vi "Editor UI.vi"(8 "error in (no error)":errorcluster, 11 "Entity Editor in":refnum<class "Entity Editor.lvclass">) -> (0 "error out":errorcluster, 3 "Entity Editor out":refnum<class "Entity Editor.lvclass">)   [LabVIEW 2020, in "Conditum-Tools.lvlib" / "Entity Editor.lvclass"]
uses:
  Entity Editor.lvclass
  Conditum/Columns/Type/Type.lvclass
  Conditum/Entity/Entity.lvclass
  ColumnPanel/ColumnPanel.lvclass
  C:/Program Files (x86)/National Instruments/LabVIEW 2020/vi.lib/IlluminatedG/IG OOPanel/OOPanel/ArrayPanel/ArrayPanel.lvclass
  Conditum/Columns/Type/Type.lvclass/Type.ctl
  <vilib>/IlluminatedG/IG OOPanel/OOPanel/ArrayManager/ArrayManager.lvclass
  2443108f-0f49-4029-b3c0-d61e9c764f54.vi
  1c4234d0-757c-494a-9175-61bb4fd4687c.vi
  <vilib>/Utility/LVClass/Get LV Class Name.vi
  <vilib>/Comparison/Equal/Equal Functor/Equal Functor.lvclass
panel:
  in  "Reset Entity":bool
  in  "Save Entity":bool
  in  "Fields":i32(listbox)
  out "Definition":refnum<class "Type.lvclass">[](array[class])
  out "Target Entity Paths":path[](array[path])
  in  "Refresh Targets":bool
  in  "Target":string(combo)
  in  "Refresh Projects":bool
  in  "New Entity":bool
  in  "Remove Field":bool
  in  "Add Field":bool
  in  "Entities":i32(listbox)
  in  "Project":string(combo)
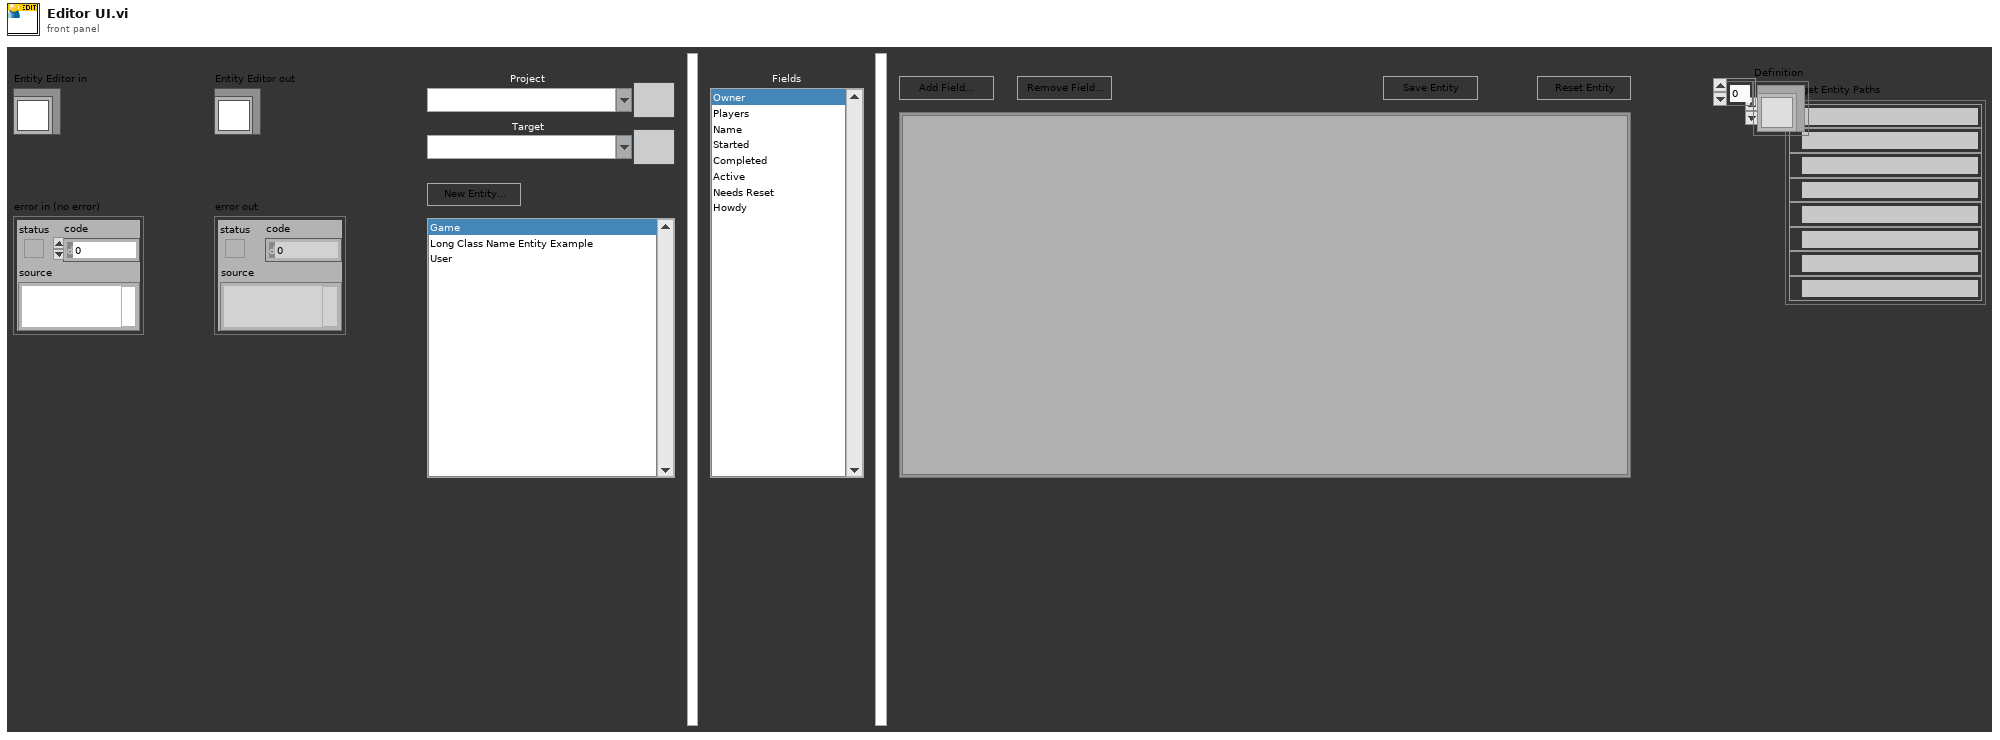
[diagram p1: front panel]
types:
  T1 = typedef "Conditum.lvlib/Field Type.ctl" = enum16{"None", "ID", "Boolean", "Integer", "Double", "Timestamp", "String", "Text", "Entity"}
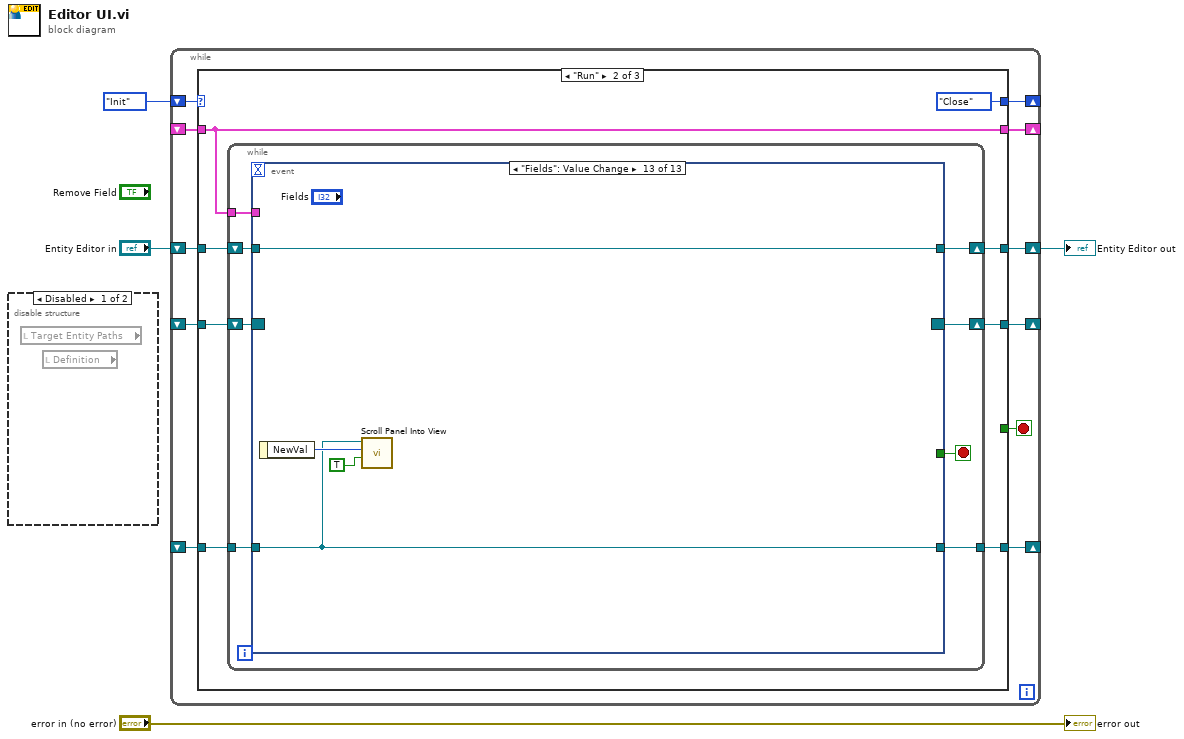
[diagram p0: block diagram]
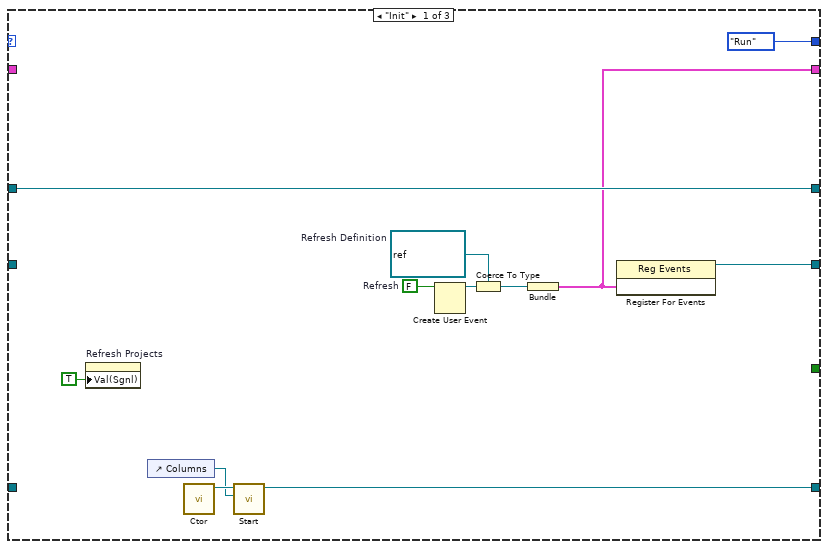
[diagram p3: hidden frame]
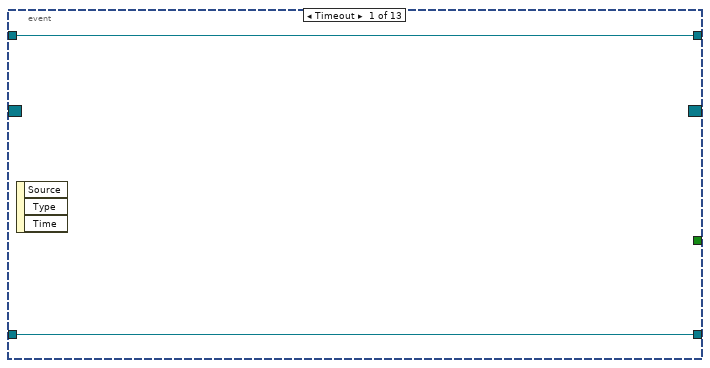
[diagram p4: hidden frame]
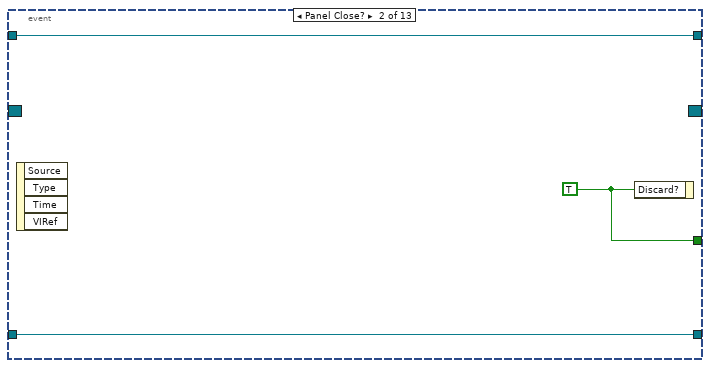
[diagram p5: hidden frame]
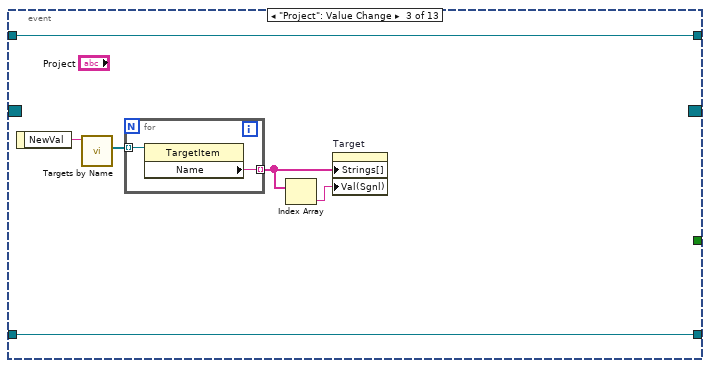
[diagram p6: hidden frame]
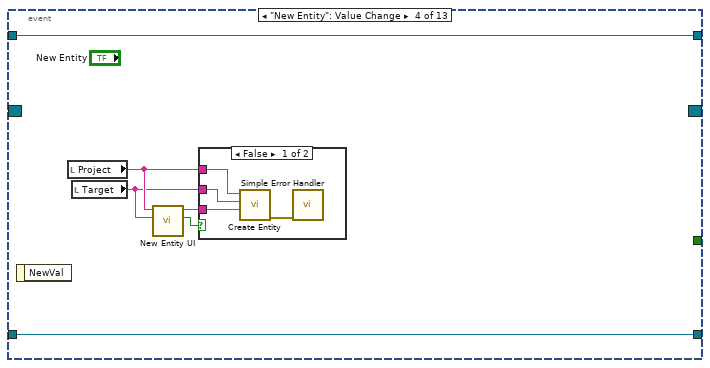
[diagram p7: hidden frame]
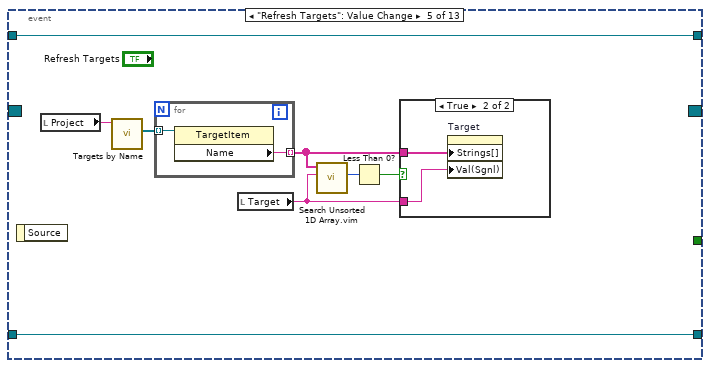
[diagram p9: hidden frame]
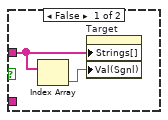
[diagram p10: hidden frame]
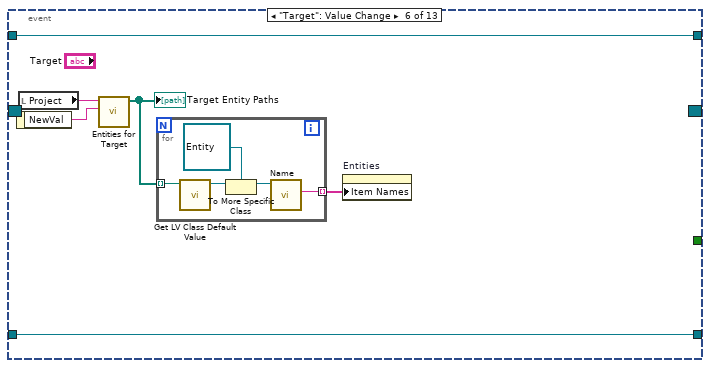
[diagram p11: hidden frame]
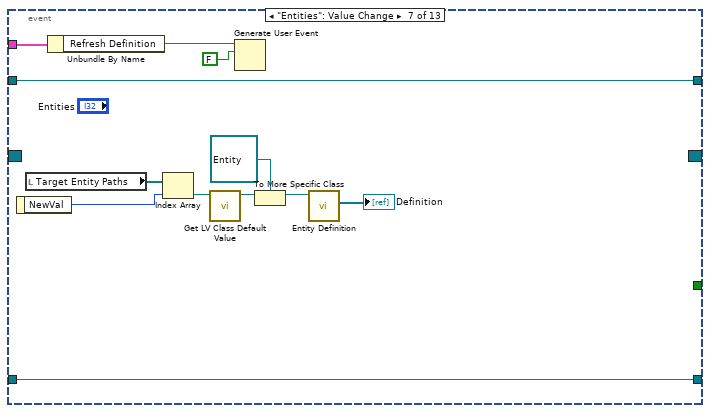
[diagram p12: hidden frame]
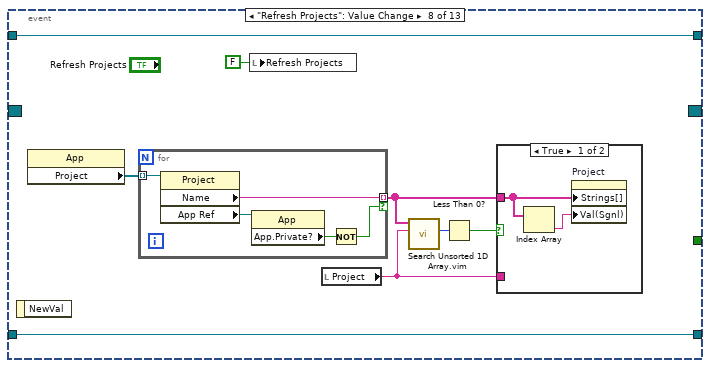
[diagram p13: hidden frame]
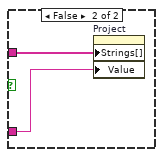
[diagram p14: hidden frame]
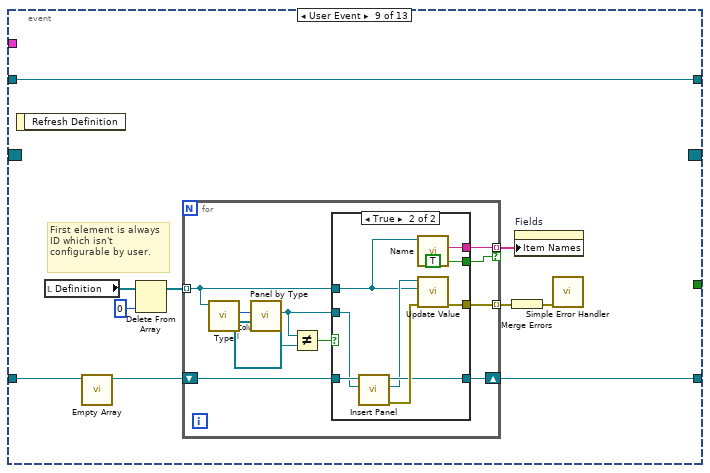
[diagram p15: hidden frame]
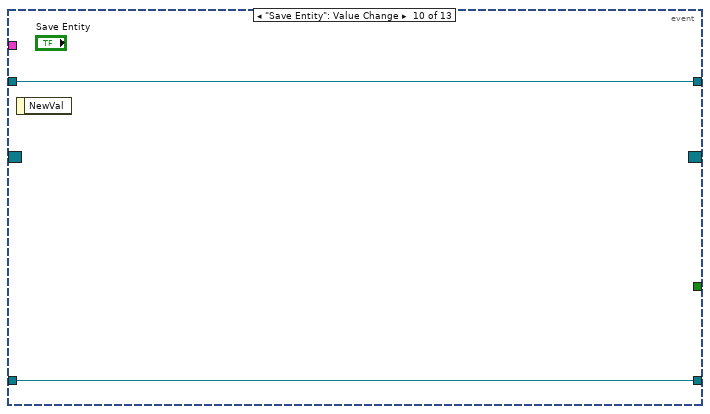
[diagram p17: hidden frame]
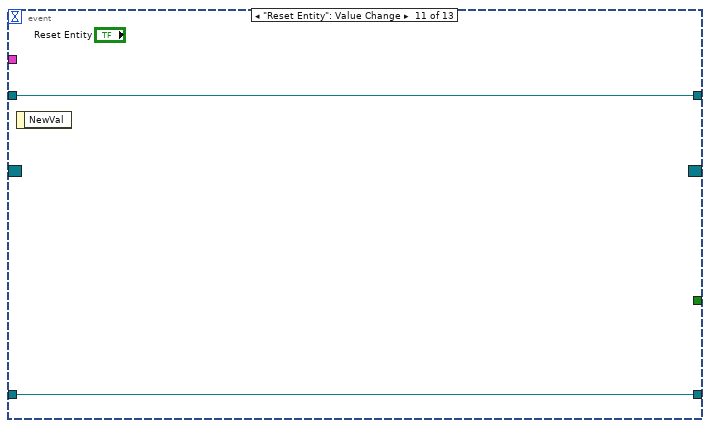
[diagram p18: hidden frame]
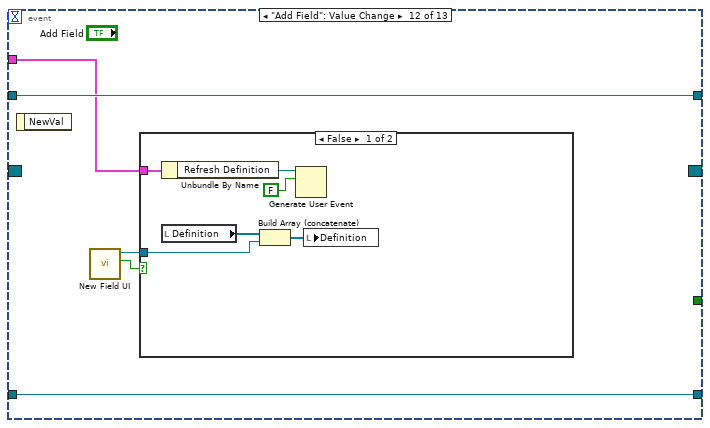
[diagram p19: hidden frame]
diagram:
  n1 = disable-structure shown="Disabled" {
    frame Disabled {
      n2 = local read "Target Entity Paths"() -> ()  [unwired: 1 out]
      n3 = local read "Definition"() -> ()  [unwired: 1 out]
    }
    frame Enabled {
    }
  }
  n4 = while {
    shift-right: [w14] -> _
    shift-left: enum16{"Init", "Run", "Close"}."Init" ("Basic UI State") -> [w15]
    shift-right: [w12] -> w2
    shift-left: "Entity Editor in" -> [w13]
    shift-right: [w10] -> _
    shift-left: _ -> [w9]
    shift-right: [w8] -> _
    shift-left: _ -> [w7]
    shift-right: [w6] -> _
    shift-left: _ -> [w5]
    stop <- w11 stop-if-true
    n5 = case shown="\"Run\"" w15 {
      selector: w15 -> [_ _ w178]
      tunnel: [enum16{"Init", "Run", "Close"}."Run" ("Basic UI State") enum16{"Init", "Run", "Close"}."Close" ("Basic UI State") w178] -> w14
      tunnel: w13 -> [w26 w34 w177]
      tunnel: [w26 w33 w177] -> w12
      tunnel: [_ _ TRUE] -> w11
      tunnel: [w19 w31 refnum<class "ArrayManager.lvclass"> refnum ("ArrayManager out")] -> w10
      tunnel: w9 -> [_ w32 w175]
      tunnel: [w17 w29 refnum<event-registration> refnum ("Event Registration Refnum")] -> w8
      tunnel: w7 -> [_ w30 w171]
      tunnel: [w16 w28 _] -> w6
      tunnel: w5 -> [_ w28 w173]
      frame "Init" {
        w21 = refnum<user-event> refnum  # Refresh Definition
        w23 = FALSE  # Refresh
        n6 = property on="Refresh Projects" class="Bool (strict)"("Val(Sgnl)"=TRUE ("Value (Signaling)")) -> ()  [unwired: 2 in, 2 out]
        n7 = control-ref of="Columns"() -> (w24:refnum<vi>)
        n8 = call <vilib>:"Ctor.vi"() -> ("PanelArray"=w25:refnum<class "ArrayManager.lvclass">)  [unwired: 10 in, 1 out]
        n9 = call <vilib>:"Start.vi"("Container"=w24, "ArrayManager in"=w25) -> ("ArrayManager out"=w19:refnum<class "ArrayManager.lvclass">)  [unwired: 8 in, 1 out]
        n10 = Create User Event(user event datatype=w23) -> (user event=w22:refnum<user-event>)  [unwired: 1 in, 1 out]
        n11 = Coerce To Type(0:w22, 1:w21) -> (2:w20:refnum<user-event>)
        n12 = Bundle("Refresh Definition"=w20) -> (w16:cluster{"Refresh Definition":refnum<user-event>})  [unwired: 1 in]
        n13 = register-events(w16) -> (reference out=w17:refnum<event-registration>)  [unwired: 2 in, 1 out]
      }
      frame "Run" {
        n14 = while {
          shift-right: [w43] -> w33
          shift-left: w34 -> [w42]
          tunnel: w32 -> [w40]
          tunnel: [w39] -> w31
          shift-right: [w37] -> w29
          shift-left: w30 -> [w38]
          tunnel: w28 -> [w36]
          stop <- w41 stop-if-true
          n15 = event shown="[12] \"Fields\": Value Change" {
            selector: w38 -> [_ _ _ _ _ _ _ _ _ _ _ _ _]
            dyn-events: [_ _ _ _ _ _ _ _ _ _ _ _ _] -> w37
            timeout: _ -> [_ _ _ _ _ _ _ _ _ _ _ _ _]
            tunnel: [w45 w48 w54 w57 w74 w86 w103 w111 w130 w152 w154 w156 w169] -> w43
            tunnel: w42 -> [w45 w48 w54 w57 w74 w86 w103 w111 w130 w152 w154 w156 w169]
            tunnel: [_ w47 _ _ _ _ _ _ _ _ _ _ _] -> w41
            tunnel: w40 -> [w44 w46 w53 w62 w73 w85 w102 w110 w126 w151 w153 w159 w167]
            tunnel: [w44 w46 w53 w62 w73 w85 w102 w110 w124 w151 w153 w159 w167] -> w39
            tunnel: w36 -> [_ _ _ _ _ _ w94 _ _ _ _ w155 _]
            event Timeout {
              n16 = event-data() -> ()  [unwired: 1 in, 3 out]
            }
            event Panel Close? {
              w47 = TRUE ("Discard?")
              n17 = event-data() -> ()  [unwired: 1 in, 4 out]
              n18 = event-data("Discard?"=w47) -> ()  [unwired: 1 in, 1 out]
            }
            event "Project": Value Change {
              n19 = event-data() -> ("NewVal"=w52:string)  [unwired: 1 in]
              n20 = call "Targets by Name.vi"("Project Name"=w52) -> ("Targets"=w51:refnum<vi>[])  [unwired: 9 in, 1 out]
              n21 = for {
                tunnel: w51 -> [w56] mode=indexing
                tunnel: [w55] -> w50 mode=indexing
                n22 = property class="TargetItem"(reference=w56) -> ("Name"=w55:string)  [unwired: 1 in, 2 out]
              }
              n23 = Index Array(array=w50) -> (element=w49:string)  [unwired: 1 in]
              n24 = property on="Target" class="CmbBox"("Strings[]"=w50, "Val(Sgnl)"=w49) -> ()  [unwired: 2 in, 2 out]
            }
            event "New Entity": Value Change {
              n25 = event-data() -> ()  [unwired: 1 in, 1 out]
              n26 = local read "Project"() -> (w59:string)
              n27 = local read "Target"() -> (w58:string)
              n28 = call "New Entity UI.vi"("Target Name"=w58, "Project Name"=w59) -> ("Cancelled"=w61:bool, "Entity Name"=w60:string)  [unwired: 7 in, 1 out]
              n29 = case shown="False" w61 {
                tunnel: w60 -> [w66 _]
                tunnel: w59 -> [w64 _]
                tunnel: w58 -> [w65 _]
                frame False {
                  n30 = call "Create Entity.vi"("Entity Name"=w66, "Target Name"=w65, "Project Name"=w64) -> ("error out"=w63:errorcluster)  [unwired: 8 in]
                  n31 = call <vilib>:"Simple Error Handler.vi"("error in (no error)"=w63) -> ()  [unwired: 4 in, 5 out]
                }
                frame True {
                }
              }
            }
            event "Refresh Targets": Value Change {
              n32 = event-data() -> ()  [unwired: 1 in, 1 out]
              n33 = local read "Project"() -> (w71:string)
              n34 = call "Targets by Name.vi"("Project Name"=w71) -> ("Targets"=w72:refnum<vi>[])  [unwired: 9 in, 1 out]
              n35 = for {
                tunnel: w72 -> [w80] mode=indexing
                tunnel: [w79] -> w68 mode=indexing
                n36 = property class="TargetItem"(reference=w80) -> ("Name"=w79:string)  [unwired: 1 in, 2 out]
              }
              n37 = local read "Target"() -> (w67:string)
              n38 = call "Search Unsorted 1D Array.vim"("element"=w67, "unsorted 1D array"=w68) -> ("index of element"=w70:i32)  [unwired: 9 in]
              n39 = Less Than 0?(x=w70) -> (x < 0?=w69:bool)
              n40 = case shown="True" w69 {
                tunnel: w68 -> [w76 w78]
                tunnel: w67 -> [_ w77]
                frame False {
                  n41 = Index Array(array=w76) -> (element=w75:string)  [unwired: 1 in]
                  n42 = property on="Target" class="CmbBox"("Strings[]"=w76, "Val(Sgnl)"=w75) -> ()  [unwired: 2 in, 2 out]
                }
                frame True {
                  n43 = property on="Target" class="CmbBox"("Strings[]"=w78, "Val(Sgnl)"=w77) -> ()  [unwired: 2 in, 2 out]
                }
              }
            }
            event "Target": Value Change {
              n44 = event-data() -> ("NewVal"=w83:string)  [unwired: 1 in]
              n45 = local read "Project"() -> (w84:string)
              n46 = call "Entities for Target.vi"("Target Name"=w83, "Project Name"=w84) -> ("Entities"=w82:path[])  [unwired: 9 in]
              "Target Entity Paths" <- w82
              n47 = for {
                tunnel: w82 -> [w91] mode=indexing
                tunnel: [w87] -> w81 mode=indexing
                n48 = call <vilib>:"Get LV Class Default Value.vi"("class path"=w91) -> ("object"=w90:refnum<class>)  [unwired: 9 in, 1 out]
                n49 = To More Specific Class(target class=refnum<class "Entity.lvclass"> refnum ("Conditum:Entity"), reference=w90) -> (specific class reference=w88:refnum<class "Entity.lvclass">)  [unwired: 1 in, 1 out]
                n50 = call-dynamic "Name.vi"("Entity in"=w88) -> ("Name"=w87:string)  [unwired: 10 in]
              }
              n51 = property on="Entities" class="LstBox (strict)"("Item Names"=w81) -> ()  [unwired: 2 in, 2 out]
            }
            event "Entities": Value Change {
              n52 = event-data() -> ("NewVal"=w100:i32)  [unwired: 1 in]
              n53 = local read "Target Entity Paths"() -> (w101:path[])
              n54 = Unbundle By Name(w94) -> ("Refresh Definition"=w93:refnum<user-event>)
              n55 = Index Array(array=w101, index=w100) -> (element=w99:path)
              n56 = call <vilib>:"Get LV Class Default Value.vi"("class path"=w99) -> ("object"=w98:refnum<class>)  [unwired: 9 in, 1 out]
              n57 = Generate User Event(user event=w93, event data cluster=FALSE ("event data")) -> ()  [unwired: 2 in, 2 out]
              n58 = To More Specific Class(target class=refnum<class "Entity.lvclass"> refnum ("Conditum:Entity"), reference=w98) -> (specific class reference=w96:refnum<class "Entity.lvclass">)  [unwired: 1 in, 1 out]
              n59 = call "Entity Definition.vi"("Entity in"=w96) -> ("Definition"=→"Definition":refnum<class "Type.lvclass">[])  [unwired: 10 in]
            }
            event "Refresh Projects": Value Change {
              n60 = event-data() -> ()  [unwired: 1 in, 1 out]
              n61 = property class="App"() -> ("Project"=w108:refnum<vi>[])  [unwired: 2 in, 2 out]
              n62 = for {
                tunnel: w108 -> [w120] mode=indexing
                tunnel: [w117] -> w107 mode=indexing if=w116
                n63 = property class="Project"(reference=w120) -> ("Name"=w117:string, "App Ref"=w119:refnum<vi>)  [unwired: 1 in, 2 out]
                n64 = property class="App"(reference=w119) -> ("App.Private?"=w118:bool)  [unwired: 1 in, 2 out]
                n65 = Not(x=w118) -> (.not. x?=w116:bool)
              }
              n66 = local write "Refresh Projects"(FALSE ("Refresh Projects")) -> ()
              n67 = local read "Project"() -> (w104:string)
              n68 = call "Search Unsorted 1D Array.vim"("element"=w104, "unsorted 1D array"=w107) -> ("index of element"=w106:i32)  [unwired: 9 in]
              n69 = Less Than 0?(x=w106) -> (x < 0?=w105:bool)
              n70 = case shown="True" w105 {
                tunnel: w107 -> [w113 w115]
                tunnel: w104 -> [_ w114]
                frame True {
                  n71 = Index Array(array=w113) -> (element=w112:string)  [unwired: 1 in]
                  n72 = property on="Project" class="CmbBox"("Strings[]"=w113, "Val(Sgnl)"=w112) -> ()  [unwired: 2 in, 2 out]
                }
                frame False {
                  n73 = property on="Project" class="CmbBox"("Strings[]"=w115, "Value"=w114) -> ()  [unwired: 2 in, 2 out]
                }
              }
            }
            event User Event {
              # "First element is always ID which isn't configurable by user."
              n74 = event-data() -> ()  [unwired: 1 in, 1 out]
              n75 = local read "Definition"() -> (w129:refnum<class "Type.lvclass">[])
              n76 = call <vilib>:"Empty Array.vi"("ArrayManager in"=w126) -> ("ArrayManager out"=w125:refnum<class "ArrayManager.lvclass">)  [unwired: 9 in, 1 out]
              n77 = Delete From Array(array=w129, index=0) -> (array with subset deleted=w128:refnum<class "Type.lvclass">[])  [unwired: 1 in, 1 out]
              n78 = for {
                tunnel: w128 -> [w135] mode=indexing
                shift-right: [w134] -> w124
                shift-left: w125 -> [w138]
                tunnel: [w133] -> w123 mode=indexing
                tunnel: [w132] -> w121 mode=indexing if=w131
                n79 = call "Type.vi"("Type in"=w135) -> ("Type"=w140:T1)  [unwired: 10 in]
                n80 = call "Panel by Type.vi"("Type"=w140) -> ("ColumnPanel"=w136:refnum<class "ColumnPanel.lvclass">)  [unwired: 10 in]
                n81 = Not Equal?(x=w136, y=refnum<class "ColumnPanel.lvclass"> refnum) -> (x != y?=w137:bool)
                n82 = case shown="True" w137 {
                  tunnel: w138 -> [w141 w149]
                  tunnel: w136 -> [_ w148]
                  tunnel: w135 -> [_ w144]
                  tunnel: [w141 w147] -> w134
                  tunnel: [_ w146] -> w133
                  tunnel: [_ w143] -> w132
                  tunnel: [_ TRUE] -> w131
                  frame False {
                  }
                  frame True {
                    n83 = call <vilib>:"Insert Panel.vi"("Panel/Type"=w148, "PanelArray in"=w149) -> ("error out"=w150:errorcluster, "Panel"=w145:refnum<class "ColumnPanel.lvclass">, "PanelArray out"=w147:refnum<class "ArrayManager.lvclass">)  [unwired: 7 in]
                    n84 = call "Name.vi"("Type in"=w144) -> ("Table Name"=w143:string)  [unwired: 10 in]
                    n85 = call "Update Value.vi"("error in (no error)"=w150, "Type Value"=w144, "ColumnPanel in"=w145) -> ("error out"=w146:errorcluster)  [unwired: 7 in, 1 out]
                  }
                }
              }
              n86 = Merge Errors(w123) -> (w122:errorcluster)
              n87 = property on="Fields" class="LstBox (strict)"("Item Names"=w121) -> ()  [unwired: 2 in, 2 out]
              n88 = call <vilib>:"Simple Error Handler.vi"("error in (no error)"=w122) -> ()  [unwired: 4 in, 5 out]
            }
            event "Save Entity": Value Change {
              n89 = event-data() -> ()  [unwired: 1 in, 1 out]
            }
            event "Reset Entity": Value Change {
              n90 = event-data() -> ()  [unwired: 1 in, 1 out]
            }
            event "Add Field": Value Change {
              n91 = event-data() -> ()  [unwired: 1 in, 1 out]
              n92 = call "New Field UI.vi"() -> ("Cancelled"=w158:bool, "Field"=w157:refnum<class "Type.lvclass">)  [unwired: 10 in]
              n93 = case shown="False" w158 {
                tunnel: w157 -> [w164 _]
                tunnel: w155 -> [w162 _]
                frame False {
                  n94 = Unbundle By Name(w162) -> ("Refresh Definition"=w161:refnum<user-event>)
                  n95 = local read "Definition"() -> (w165:refnum<class "Type.lvclass">[])
                  n96 = Build Array (concatenate)(w165, w164) -> (w163:refnum<class "Type.lvclass">[])
                  n97 = Generate User Event(user event=w161, event data cluster=FALSE ("event data")) -> ()  [unwired: 2 in, 2 out]
                  n98 = local write "Definition"(w163) -> ()
                }
                frame True {
                }
              }
            }
            event "Fields": Value Change {
              n99 = event-data() -> ("NewVal"=w168:i32)  [unwired: 1 in]
              n100 = call <vilib>:"Scroll Panel Into View.vi"("Highlight (F)"=TRUE, "Panel Index"=w168, "ArrayManager in"=w167) -> ()  [unwired: 7 in, 2 out]
            }
          }
        }
      }
      frame "Close" {
        n101 = Unregister For Events(event registration refnum=w171) -> ()  [unwired: 1 in, 1 out]
        n102 = call <vilib>:"Cleanup.vi"("PanelArray in"=w175) -> ()  [unwired: 10 in, 1 out]
        n103 = Unbundle By Name(w173) -> ("Refresh Definition"=w172:refnum<user-event>)
        n104 = Destroy User Event(user event=w172) -> ()  [unwired: 1 in, 1 out]
      }
    }
  }
  "Entity Editor out" <- w2
  "error out" <- "error in (no error)"
